vi "Read Strings.vi"(8 "error in (no error)":errorcluster, 10 "Ctl Refnum":refnum<vi>, 11 "Worksheet Reference":refnum<k7>) -> (0 "error out":errorcluster)   [LabVIEW 2015]
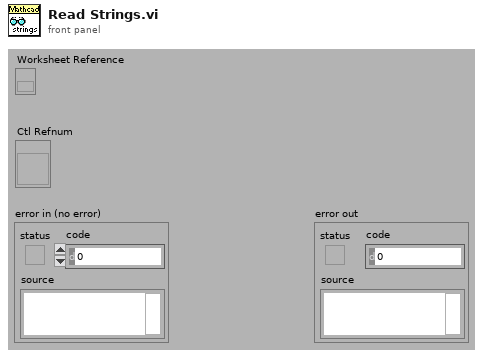
[diagram p1: front panel]
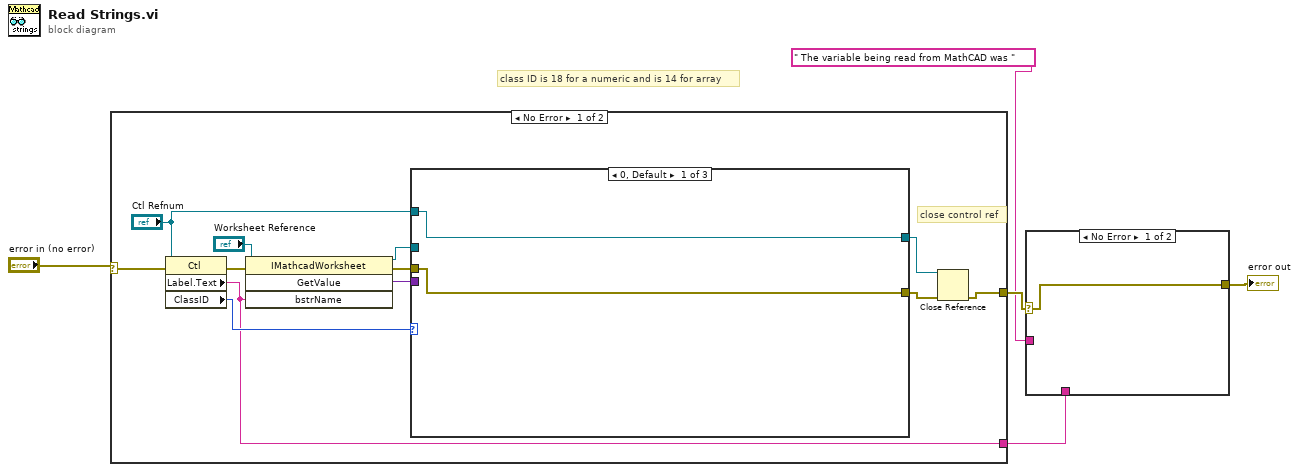
[diagram p0: block diagram]
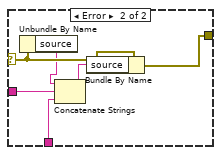
[diagram p2: hidden frame]
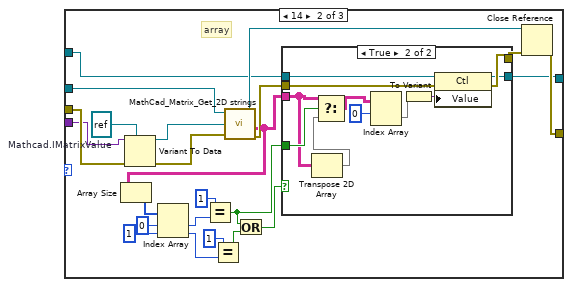
[diagram p3: hidden frame]
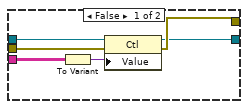
[diagram p4: hidden frame]
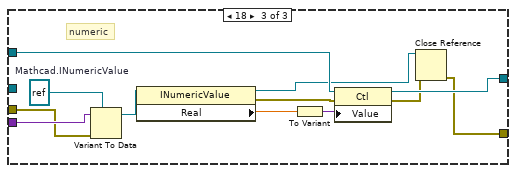
[diagram p5: hidden frame]
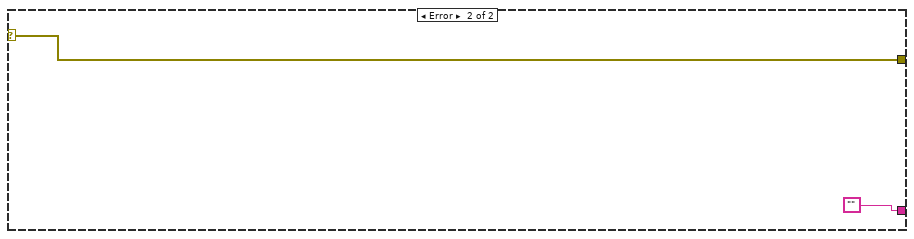
[diagram p6: hidden frame]
diagram:
  # "class ID is 18 for a numeric and is 14 for array"
  n1 = case shown="No Error" "error in (no error)" {
    selector: "error in (no error)" -> [w16 w73]
    tunnel: [w8 w73] -> w4
    tunnel: [w6 ""] -> w2
    frame No Error {
      # "close control ref"
      n2 = property class="Ctl"(reference="Ctl Refnum", error in=w16) -> (error out=w15:errorcluster, "Label.Text"=w6:string, "ClassID"=w14:u32)  [unwired: 1 out]
      n3 = invoke class="IMathcadWorksheet" method="GetValue"(reference="Worksheet Reference", error in=w15, "bstrName"=w6) -> (reference out=w11:refnum<k7>, error out=w12:errorcluster, "GetValue"=w13:variant)  [unwired: 1 in, 1 out]
      n4 = case shown="0, Default" w14 {
        tunnel: [w19 w32 w68] -> w7
        tunnel: w13 -> [_ w41 w67]
        tunnel: w12 -> [w18 w42 w66]
        tunnel: w11 -> [_ w38 _]
        tunnel: "Ctl Refnum" -> [w19 w20 w63]
        tunnel: [w18 w37 w60] -> w9
        frame 0, Default {
        }
        frame 14 {
          w40 = refnum<k7> refnum  # Mathcad.IMatrixValue
          # "array"
          n5 = Variant To Data(error in=w42, type=w40, Variant=w41) -> (data=w39:refnum<k7>, error out=w33:errorcluster)
          n6 = call "MathCad_Matrix_Get_2D strings.vi"("Worksheet Reference"=w38, "Mathcad.IMatrixValue Refnum"=w39, "error out 2"=w33) -> ("Mathcad.IMatrixValue Refnum"=w36:refnum<k7>, "Array"=w31:string[][], "error out"=w35:errorcluster)  [unwired: 1 out]
          n7 = Array Size(array=w31) -> (size(s)=w30:i32[])
          n8 = Index Array(array=w30, index #1=0 ("index"), index #2=1 ("index")) -> (element #1=w27:i32, element #2=w24:i32)
          n9 = Equal?(x=1 ("index"), y=w27) -> (x = y?=w21:bool)
          n10 = Equal?(x=1 ("index"), y=w24) -> (x = y?=w23:bool)
          n11 = Or(x=w21, y=w23) -> (x .or. y?=w22:bool)
          n12 = case shown="True" w22 {
            tunnel: w35 -> [w47 w58]
            tunnel: [w46 w57] -> w34
            tunnel: [w45 w56] -> w32
            tunnel: w20 -> [w44 w55]
            tunnel: w31 -> [w43 w50]
            tunnel: w21 -> [_ w52]
            frame False {
              n13 = To Variant(anything=w43) -> (Variant=w48:variant)
              n14 = property class="Ctl"(reference=w44, error in=w47, "Value"=w48) -> (reference out=w45:refnum<vi>, error out=w46:errorcluster)
            }
            frame True {
              n15 = Transpose 2D Array(2D array=w50) -> (transposed array=w49:string[][])
              n16 = Select(t=w50, s=w52, f=w49) -> (s? t:f=w51:string[][])
              n17 = Index Array(array=w51, index (row)=0) -> (element=w54:string[])  [unwired: 1 in]
              n18 = To Variant(anything=w54) -> (Variant=w59:variant)
              n19 = property class="Ctl"(reference=w55, error in=w58, "Value"=w59) -> (reference out=w56:refnum<vi>, error out=w57:errorcluster)
            }
          }
          n20 = Close Reference(reference=w36, error in (no error)=w34) -> (error out=w37:errorcluster)
        }
        frame 18 {
          w65 = refnum<k7> refnum  # Mathcad.INumericValue
          # "numeric"
          n21 = Variant To Data(error in=w66, type=w65, Variant=w67) -> (data=w64:refnum<k7>)  [unwired: 1 out]
          n22 = property class="INumericValue"(reference=w64) -> (reference out=w62:refnum<k7>, error out=w69:errorcluster, "Real"=w71:dbl)  [unwired: 1 in]
          n23 = To Variant(anything=w71) -> (Variant=w70:variant)
          n24 = property class="Ctl"(reference=w63, error in=w69, "Value"=w70) -> (reference out=w68:refnum<vi>, error out=w61:errorcluster)
          n25 = Close Reference(reference=w62, error in (no error)=w61) -> (error out=w60:errorcluster)
        }
      }
      n26 = Close Reference(reference=w7, error in (no error)=w9) -> (error out=w8:errorcluster)
    }
    frame Error {
    }
  }
  n27 = case shown="No Error" w4 {
    selector: w4 -> [w74 w80]
    tunnel: [w74 w75] -> w3
    tunnel: w2 -> [_ w77]
    tunnel: " The variable being read from MathCAD was " ("string") -> [_ w76]
    frame No Error {
    }
    frame Error {
      n28 = Unbundle By Name(w80) -> ("source"=w79:string)
      n29 = Concatenate Strings(w79, w76, w77) -> (w78:string)
      n30 = Bundle By Name(cluster=w80, "source"=w78) -> (w75:errorcluster)
    }
  }
  "error out" <- w3
